vi "Initialize People Tracking Refs.vi"(8 "error in (no error)":errorcluster) -> (0 "error out":errorcluster, 3 "ball tracking refs":T7={"acquired image"=refnum, "threshold image"=refnum, "Video Handle out"=0, "Kinect Handle"=0, "Video and Depth config"={"Video Resolution"=enum."FREENECT_RESOLUTION_LOW", "Video Format"=enum."FREENECT_VIDEO_RGB", "Depth Format"=enum."FREENECT_DEPTH_11BIT", "Depth Resolution"=enum."FREENECT_RESOLUTION_MEDIUM"}})   [LabVIEW 2014]
doc: "Creates image buffers and initializes a camera session. This VI outputs a cluster containing the camera session and image references for use by other sub VIs."
uses:
  Ball Tracking Image Refs.ctl
  <vilib>/vision/Image Controls.llb/IMAQ Image.ctl
  KinectProject/subVIs/Video Resolution Control.ctl
  KinectProject/subVIs/Video Format Control.ctl
  KinectProject/subVIs/Depth Format Control.ctl
  KinectProject/subVIs/Depth Resolution Control.ctl
  KinectProject/subVIs/Led Control.ctl
  KinectProject/subVIs/Log Level Control.ctl
panel:
  in  "Led Option":T1
  in  "tilt degree":i32
  in  "Video and Depth config":T6={"Video Resolution"=enum."FREENECT_RESOLUTION_MEDIUM", "Video Format"=enum."FREENECT_VIDEO_RGB", "Depth Format"=enum."FREENECT_DEPTH_11BIT", "Depth Resolution"=enum."FREENECT_RESOLUTION_MEDIUM"}
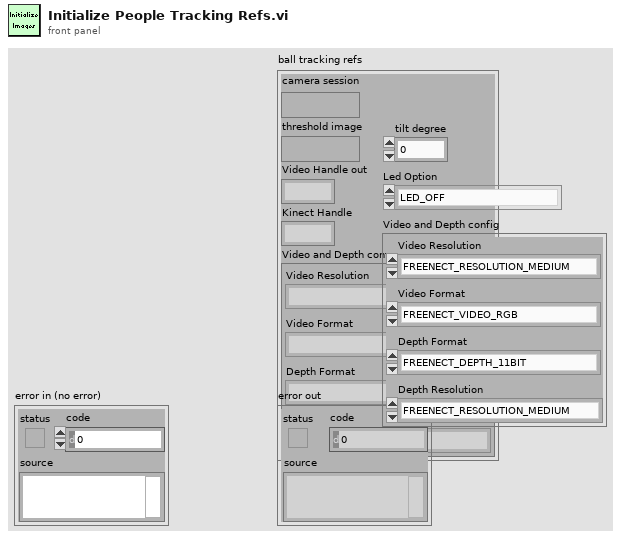
[diagram p1: front panel]
types:
  T1 = typedef "Led Control.ctl" = enum32{"LED_OFF", "LED_GREEN", "LED_RED", "LED_YELLOW", "LED_BLINK_GREEN", "LED_BLINK_GREEN2", "LED_BLINK_RED_YELLOW"}
  T2 = typedef "Video Resolution Control.ctl" = enum32{"FREENECT_RESOLUTION_LOW", "FREENECT_RESOLUTION_MEDIUM", "FREENECT_RESOLUTION_HIGH"}
  T3 = typedef "Video Format Control.ctl" = enum32{"FREENECT_VIDEO_RGB", "FREENECT_VIDEO_BAYER", "FREENECT_VIDEO_IR_8BIT", "FREENECT_VIDEO_IR_10BIT", "FREENECT_VIDEO_IR_10BIT_PACKED", "FREENECT_VIDEO_YUV_RGB", "FREENECT_VIDEO_YUV_RAW"}
  T4 = typedef "Depth Format Control.ctl" = enum32{"FREENECT_DEPTH_11BIT", "FREENECT_DEPTH_10BIT", "FREENECT_DEPTH_11BIT_PACKED", "FREENECT_DEPTH_10BIT_PACKED", "FREENECT_DEPTH_REGISTERED", "FREENECT_DEPTH_MM"}
  T5 = typedef "Depth Resolution Control.ctl" = enum16{"FREENECT_RESOLUTION_TINY", "FREENECT_RESOLUTION_LOW", "FREENECT_RESOLUTION_MEDIUM"}
  T6 = cluster{"Video Resolution":T2, "Video Format":T3, "Depth Format":T4, "Depth Resolution":T5}
  T7 = typedef "Ball Tracking Image Refs.ctl" = cluster{"acquired image":T8, "threshold image":T8, "Video Handle out":i64, "Kinect Handle":i64, "Video and Depth config":cluster{"Video Resolution":T2, "Video Format":T3, "Depth Format":T4, "Depth Resolution":T5}}
  T8 = typedef "IMAQ Image.ctl" = refnum<image>
  T9 = typedef "Log Level Control.ctl" = enum32{"FREENECT_LOG_FATAL", "FREENECT_LOG_ERROR", "FREENECT_LOG_WARNING", "FREENECT_LOG_NOTICE", "FREENECT_LOG_INFO", "FREENECT_LOG_DEBUG", "FREENECT_LOG_SPEW", "FREENECT_LOG_FLOOD"}
  T10 = typedef "Image Type" = u32
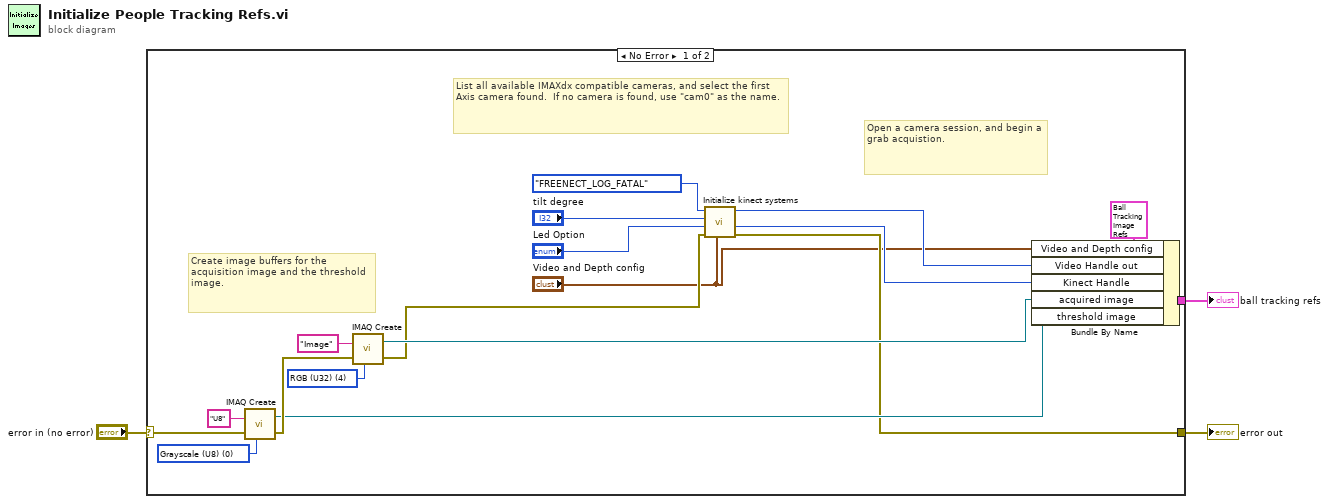
[diagram p0: block diagram]
diagram:
  n1 = case shown="No Error" "error in (no error)" {
    selector: "error in (no error)" -> [w12 w22]
    tunnel: [w13 _] -> w3
    tunnel: [w7 w22] -> w1
    frame No Error {
      w21 = T10 0 items=["Grayscale (U8)", "Grayscale (I16)", "Grayscale (SGL)", "Complex (CSG)", "RGB (U32)", "HSL (U32)", "RGB (U64)", "Grayscale (U16)"] ("Image Type")
      w19 = T10 4 items=["Grayscale (U8)", "Grayscale (I16)", "Grayscale (SGL)", "Complex (CSG)", "RGB (U32)", "HSL (U32)", "RGB (U64)", "Grayscale (U16)"] ("Image Type")
      # "List all available IMAXdx compatible cameras, and select the first Axis camera found.  If no camera is found, use \"cam0\" as the name."
      # "Create image buffers for the acquisition image and the threshold image."
      # "Open a camera session, and begin a grab acquistion."
      n2 = call "IMAQ Create"("Image Name"="U8", "Image Type"=w21, "error in (no error)"=w12) -> ("New Image"=w14:T8, "error out"=w16:errorcluster)  [unwired: 2 in]
      n3 = call "IMAQ Create"("Image Name"="Image", "Image Type"=w19, "error in (no error)"=w16) -> ("New Image"=w15:T8, "error out"=w8:errorcluster)  [unwired: 2 in]
      n4 = call "Initialize kinect systems.vi"("Video and Depth config"="Video and Depth config", "error in (no error)"=w8, "Led Option"="Led Option", "tilt degree"="tilt degree", "Log Level"=Log_Level_Control."FREENECT_LOG_FATAL") -> ("error out"=w7:errorcluster, "Kinect Handle"=w5:i64, "Video Handle out"=w6:i64)  [unwired: 3 in, 1 out]
      n5 = Bundle By Name(cluster=T7 {"acquired image"=refnum, "threshold image"=refnum, "Video Handle out"=0, "Kinect Handle"=0, "Video and Depth config"={"Video Resolution"=enum."FREENECT_RESOLUTION_LOW", "Video Format"=enum."FREENECT_VIDEO_RGB", "Depth Format"=enum."FREENECT_DEPTH_11BIT", "Depth Resolution"=enum."FREENECT_RESOLUTION_MEDIUM"}} ("ball tracking refs"), "Video and Depth config"="Video and Depth config", "Video Handle out"=w6, "Kinect Handle"=w5, "acquired image"=w15, "threshold image"=w14) -> (w13:T7)
    }
    frame Error {
    }
  }
  "ball tracking refs" <- w3
  "error out" <- w1
